vi "Tear Down TS.vi"(8 "error in":errorcluster, 11 "Heat Flow Test Stand in":refnum<class "Heat Flow Test Stand.lvclass">) -> (0 "error out":errorcluster, 3 "Heat Flow Test Stand out":refnum<class "Heat Flow Test Stand.lvclass">)   [LabVIEW 2019, in "Test Stands.lvlib" / "Heat Flow Test Stand.lvclass"]
uses:
  Heat Flow Test Stand.lvclass
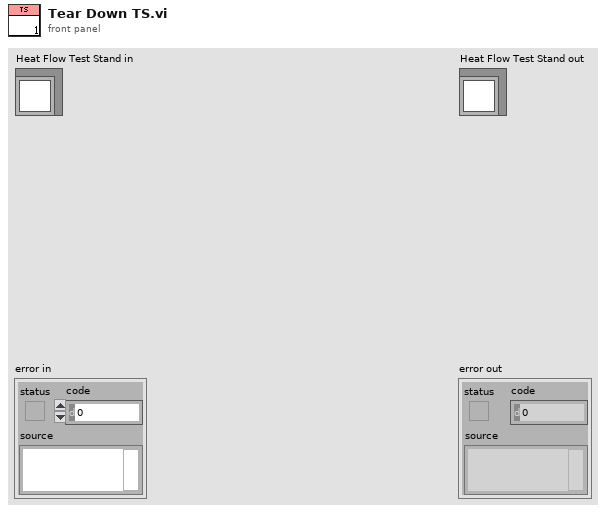
[diagram p1: front panel]
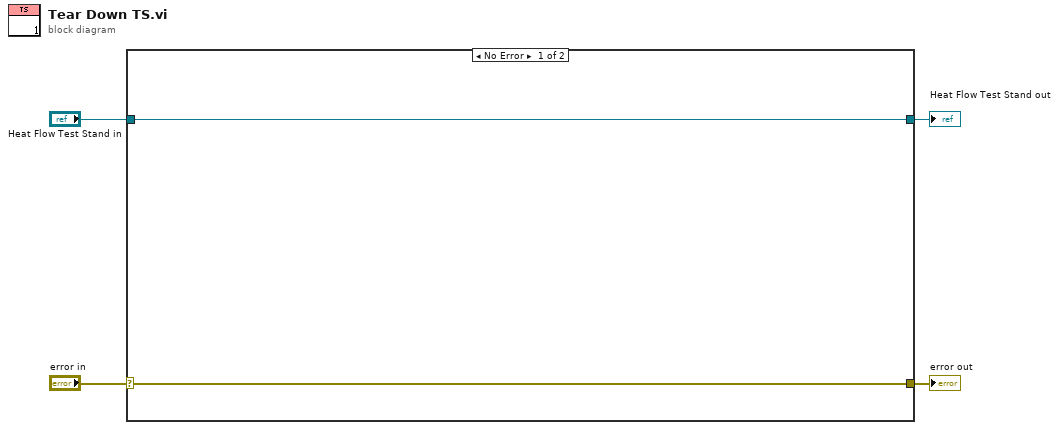
[diagram p0: block diagram]
diagram:
  n1 = case shown="No Error" "error in" {
    selector: "error in" -> [w5 w8]
    tunnel: [w5 w8] -> w4
    tunnel: [w6 w7] -> w3
    tunnel: "Heat Flow Test Stand in" -> [w6 w7]
    frame No Error {
    }
    frame Error {
    }
  }
  "error out" <- w4
  "Heat Flow Test Stand out" <- w3
